vi "Calculate Assign Pt.vi"(4 "reflective index":dbl=1.35 format="%#_13g", 5 "Zp array":dbl[][](array[numeric]), 6 "deform array":dbl[](array[numeric])=[1.0, 1.0, 1.0, 0.0, 0.0, 0.0, 0.0, 0.0, 0.0], 7 "Za array":dbl[][](array[numeric]), 8 "grid info":dbl[](array[numeric]), 9 "EyeCenter":dbl[](array[numeric])=[0.0, 5.0], 10 "EyeRadius":dbl=3.0, 11 "AssignPoint":dbl[](array[numeric])=[0.0, 5.0, 0.0]) -> (2 "insdie boundary":bool, 3 "T Cal":dbl[](array[numeric])=[0.0, 5.0, 0.0])   [LabVIEW 2010]
doc: "This VI calulates if the assigned point is out of bound or not."
uses:
  <vilib>/Analysis/NI_AALPro.lvlib
  <vilib>/Analysis/_algsub.llb/Real Vector Norm.vi
  <vilib>/Analysis/_algsub.llb/Vector Norm Type.ctl
  <vilib>/Analysis/NI_AALBase.lvlib
  <vilib>/Analysis/baseanly.llb/A x Vector.vi
  <vilib>/Analysis/Matrix/NI_Matrix.lvlib
  <vilib>/Analysis/Matrix/Numeric/Conversions/Array To Matrix - RA2.vi
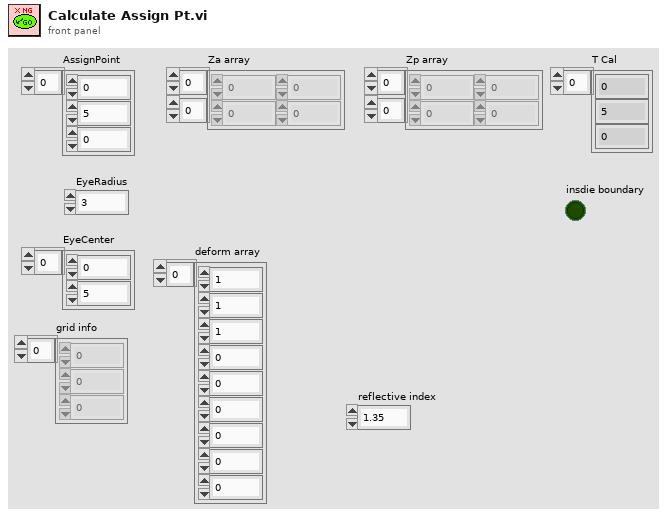
[diagram p1: front panel]
types:
  T1 = typedef "NI_AALPro.lvlib/Vector Norm Type.ctl" = u16
  T2 = typedef "NI_Matrix.lvlib/RealMatrix.ctl" = dbl[][]
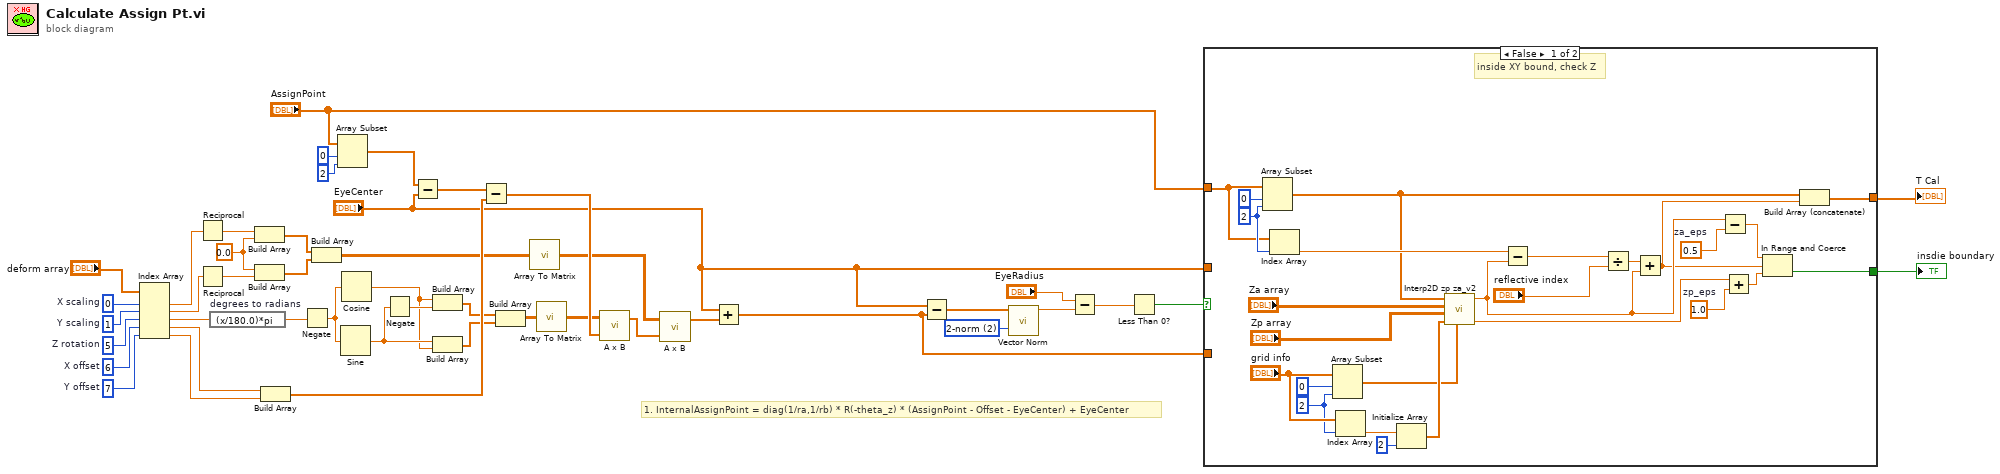
[diagram p0: block diagram]
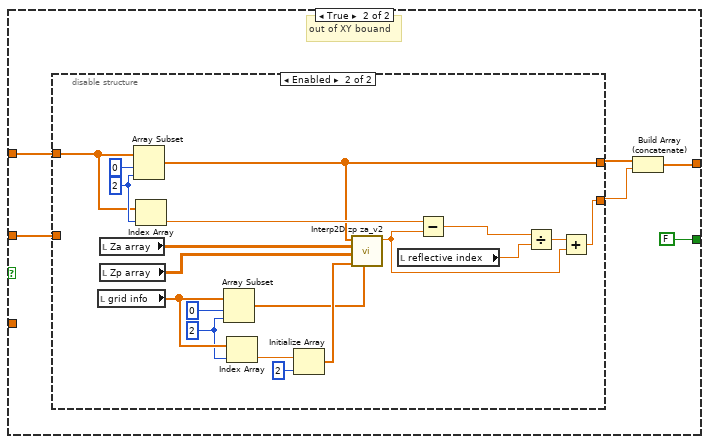
[diagram p2: hidden frame]
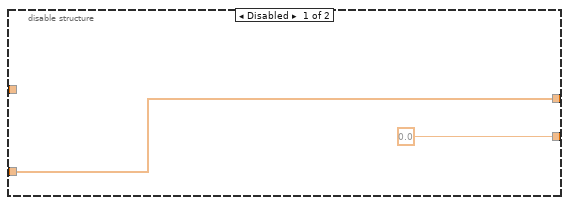
[diagram p3: hidden frame]
diagram:
  w31 = 0.0 ("element")
  w36 = 7  # Y offset
  w37 = 6  # X offset
  w38 = 5  # Z rotation
  w39 = 1  # Y scaling
  w40 = 0  # X scaling
  w45 = T1 2 items=["1-norm"=1, "2-norm"=2, "Inf-norm"=3, "-Inf-norm"=4, "User Defined"=5] ("norm type")
  # "1. InternalAssignPoint = diag(1/ra,1/rb) * R(-theta_z) * (AssignPoint - Offset - EyeCenter) + EyeCenter"
  n1 = Index Array(array="deform array", index #1=w40, index #2=w39, index #3=w38, index #4=w37, index #5=w36) -> (element #1=w35:dbl, element #2=w34:dbl, element #3=w24:dbl, element #4=w28:dbl, element #5=w27:dbl)
  n2 = Reciprocal(x=w35) -> (1/x=w32:dbl)
  n3 = Reciprocal(x=w34) -> (1/x=w33:dbl)
  n4 = expression code="(x/180.0)*pi" "degrees to radians"(w24) -> (w23:dbl)
  n5 = Build Array(w32, w31) -> (w30:dbl[])
  n6 = Build Array(w31, w33) -> (w29:dbl[])
  n7 = Build Array(w28, w27) -> (w26:dbl[])
  n8 = Negate(x=w23) -> (-x=w22:dbl)
  n9 = Build Array(w30, w29) -> (w12:dbl[][])
  n10 = Array Subset(array="AssignPoint", index=0, length=2) -> (w5:dbl[])
  n11 = Sine(x=w22) -> (sin(x)=w20:dbl)
  n12 = Cosine(x=w22) -> (cos(x)=w19:dbl)
  n13 = Negate(x=w20) -> (-x=w21:dbl)
  n14 = Subtract(x=w5, y="EyeCenter") -> (x-y=w25:dbl[])
  n15 = Build Array(w19, w21) -> (w18:dbl[])
  n16 = Build Array(w20, w19) -> (w17:dbl[])
  n17 = Subtract(x=w25, y=w26) -> (x-y=w15:dbl[])
  n18 = Build Array(w18, w17) -> (w16:dbl[][])
  n19 = call-poly <vilib>:"Array To Matrix.vi"("Real 2D Array"=w12) -> ("Real Matrix"=w11:T2)
  n20 = call-poly <vilib>:"Array To Matrix.vi"("Real 2D Array"=w16) -> ("Real Matrix"=w14:T2)
  n21 = call-poly <vilib>:"A x B.vi"("Vector"=w15, "A"=w14) -> ("A x Vector"=w13:dbl[])  [unwired: 1 out]
  n22 = call-poly <vilib>:"A x B.vi"("Vector"=w13, "A"=w11) -> ("A x Vector"=w10:dbl[])  [unwired: 1 out]
  n23 = Add(x="EyeCenter", y=w10) -> (x+y=w9:dbl[])
  n24 = Subtract(x="EyeCenter", y=w9) -> (x-y=w46:dbl[])
  n25 = call-poly <vilib>:"Vector Norm.vi"("norm type"=w45, "Input Vector"=w46) -> ("norm"=w44:dbl)  [unwired: 8 in, 1 out]
  n26 = Subtract(x="EyeRadius", y=w44) -> (x-y=w8:dbl)
  n27 = Less Than 0?(x=w8) -> (x < 0?=w43:bool)
  n28 = case shown="False" w43 {
    tunnel: w9 -> [_ _]
    tunnel: "AssignPoint" -> [w67 w73]
    tunnel: [w60 FALSE] -> w4
    tunnel: [w51 w77] -> w2
    tunnel: "EyeCenter" -> [_ w75]
    frame False {
      w54 = 0.5  # za_eps
      w55 = 1.0  # zp_eps
      w68 = 2 ("length")
      w70 = 2 ("length")
      # "inside XY bound, check Z"
      n29 = Array Subset(array=w67, index=0, length=w68) -> (w52:dbl[])
      n30 = Index Array(array=w67, index=w68) -> (element=w66:dbl)
      n31 = Array Subset(array="grid info", index=0, length=w70) -> (w47:dbl[])
      n32 = Index Array(array="grid info", index=w70) -> (element=w50:dbl)
      n33 = Initialize Array(w50, 2 ("dimension size")) -> (w48:dbl[])
      n34 = call "Interp2D zp za_v2.vi"("XY Grid min"=w47, "XY Quantization Factor"=w48, "Zp array"="Zp array", "Za array"="Za array", "Tip Position"=w52) -> ("zp"=w56:dbl, "za"=w59:dbl)  [unwired: 5 in]
      n35 = Subtract(x=w66, y=w59) -> (x-y=w65:dbl)
      n36 = Divide(x=w65, y="reflective index") -> (x/y=w63:dbl)
      n37 = Add(x=w63, y=w59) -> (x+y=w53:dbl)
      n38 = Subtract(x=w59, y=w54) -> (x-y=w58:dbl)
      n39 = Add(x=w56, y=w55) -> (x+y=w57:dbl)
      n40 = In Range and Coerce(upper limit=w58, x=w53, lower limit=w57) -> (In Range?=w60:bool)  [unwired: 1 out]
      n41 = Build Array (concatenate)(w52, w53) -> (w51:dbl[])
    }
    frame True {
      # "out of XY bouand"
      n42 = disable-structure shown="Enabled" {
        disable-tunnel: [w80 w86] -> w76
        disable-tunnel: w75 -> [w80 _]
        disable-tunnel: [0.0 w87] -> w74
        disable-tunnel: w73 -> [_ w97]
        frame Disabled {
        }
        frame Enabled {
          w85 = 2 ("length")
          w98 = 2 ("length")
          n43 = local read "grid info"() -> (w92:dbl[])
          n44 = local read "Za array"() -> (w89:dbl[][])
          n45 = local read "Zp array"() -> (w90:dbl[][])
          n46 = Array Subset(array=w97, index=0, length=w98) -> (w86:dbl[])
          n47 = Index Array(array=w97, index=w98) -> (element=w88:dbl)
          n48 = Array Subset(array=w92, index=0, length=w85) -> (w81:dbl[])
          n49 = Index Array(array=w92, index=w85) -> (element=w84:dbl)
          n50 = Initialize Array(w84, 2 ("dimension size")) -> (w82:dbl[])
          n51 = call "Interp2D zp za_v2.vi"("XY Grid min"=w81, "XY Quantization Factor"=w82, "Zp array"=w90, "Za array"=w89, "Tip Position"=w86) -> ("za"=w96:dbl)  [unwired: 5 in, 1 out]
          n52 = local read "reflective index"() -> (w94:dbl)
          n53 = Subtract(x=w88, y=w96) -> (x-y=w93:dbl)
          n54 = Divide(x=w93, y=w94) -> (x/y=w95:dbl)
          n55 = Add(x=w95, y=w96) -> (x+y=w87:dbl)
        }
      }
      n56 = Build Array (concatenate)(w76, w74) -> (w77:dbl[])
    }
  }
  "insdie boundary" <- w4
  "T Cal" <- w2
